vi "OAT Easy Continuous Resampling (Digital Tach).vi"(0 "scaled signal [EU]":waveform(dbl)={"t0"=timestamp(0 s since 1904-01-01), "dt"=0.0, "Y"=[]}, 1 "reset? (True)":bool=TRUE, 7 "digital tach info":T3={"tacho counts"=[], "counter timebase [Hz]"=20000000.0, "counter task type"=enum."event counting", "counter digit (32)"=32}, 9 "pulse/revolution (1)":i32=1, 11 "error in (no error)":errorcluster, 12 "max order (auto)":i32) -> (3 "speed profile":T1 {"speed [RPM]" format="%.2f"; "time [s]" format="%.2f"}, 4 "resampled signal":cluster{"r0":dbl, "dr":dbl, "Y":dbl[]} {"r0" format="%.2p"; "dr" format="%.2p"; "Y" format="%.2f"}, 6 "unit label":string, 10 "time instant":dbl[](array[numeric]) format="%.2f", 14 "channel info":T2={"sensor sensitivity [mV/EU]"=1000.0, "engineering units"=enum."V", "dB reference [EU]"=1.0, "custom label"="EU", "weighting filter"=enum."Linear", "pregain [dB]"=0.0} {"pregain [dB]" format="%.2f"; "dB reference [EU]" format="%.1e"; "sensor sensitivity [mV/EU]" format="%.2f"}, 15 "error out":errorcluster)   [LabVIEW 2017]
doc: "Resamples the even time-sampled <B>scaled signal [EU]</B> to an even angle-sampled signal. You can use this polymorphic VI to resample an analog tachometer signal or a digital tachometer signal. The data type you wire to the <B>analog tach signal</B> input determines the polymorphic instance to use."
uses:
  <vilib>/addons/Sound and Vibration/Order Analysis/Tach Process/SubVIs/digital tach info.ctl
  <vilib>/addons/Sound and Vibration/Order Analysis/Tach Process/SubVIs/speed profile.ctl
  <vilib>/addons/Sound and Vibration/Order Analysis/Backward Compatibility/OAT Resample Waveform (Single Channel).vi
  <vilib>/addons/Sound and Vibration/Order Analysis/Tach Process/SoundVib_TachProcess.lvlib
panel:
  # "OAT Easy Continuous Resampling (Digital Tach)"
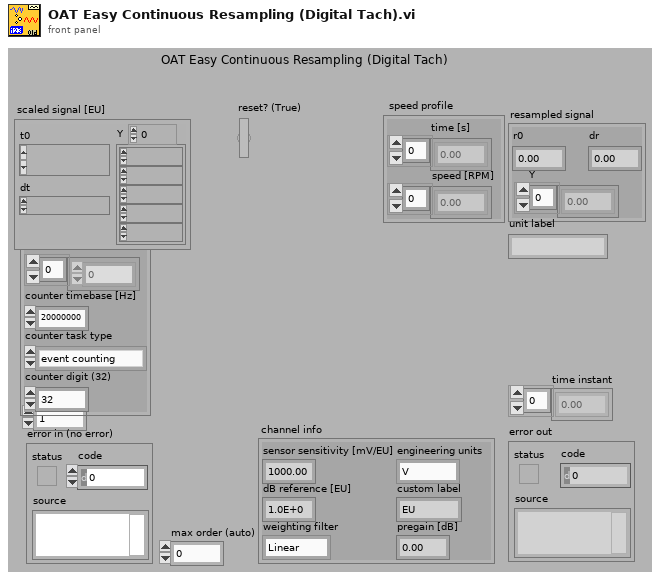
[diagram p1: front panel]
types:
  T1 = typedef "SoundVib_TachProcess.lvlib/speed profile.ctl" = cluster{"time [s]":dbl[], "speed [RPM]":dbl[]}
  T2 = cluster{"sensor sensitivity [mV/EU]":dbl, "engineering units":enum16{"custom...", "V", "Pa", "g", "m/s^2", "m/s", "m", "in/s^2", "in/s", "in"}, "dB reference [EU]":dbl, "custom label":string, "weighting filter":enum16{"Linear", "A-weighting", "B-weighting", "C-weighting"}, "pregain [dB]":dbl}
  T3 = typedef "SoundVib_TachProcess.lvlib/digital tach info.ctl" = cluster{"tacho counts":i64[], "counter timebase [Hz]":dbl, "counter task type":enum16{"period measurement", "event counting"}, "counter digit (32)":i32}
  T4 = typedef "svc_Channel Info.ctl" = cluster{"sensor sensitivity":dbl, "engineering units":T5, "dB reference":dbl, "custom label":string, "weighting filter":T6, "pregain":dbl}
  T5 = typedef "svc_Engineering Units Text Ring.ctl" = u16
  T6 = typedef "svc_Weighting Filter Text Ring.ctl" = u16
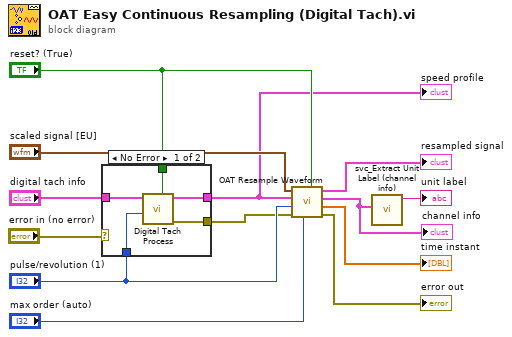
[diagram p0: block diagram]
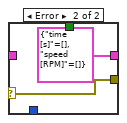
[diagram p2: hidden frame]
diagram:
  n1 = case shown="No Error" "error in (no error)" {
    selector: "error in (no error)" -> [_ w19]
    tunnel: "digital tach info" -> [w18 _]
    tunnel: "pulse/revolution (1)" -> [w17 _]
    tunnel: "reset? (True)" -> [w16 _]
    tunnel: [w15 T1 {"time [s]"=[], "speed [RPM]"=[]} ("speed profile")] -> w7
    tunnel: [w14 w19] -> w1
    frame No Error {
      n2 = call <vilib>:"Digital Tach Process.vi"("reset? (True)"=w16, "pulse/revolution (1)"=w17, "digital tach info"=w18) -> ("error out"=w14:errorcluster, "speed profile"=w15:T1)  [unwired: 6 in, 1 out]
    }
    frame Error {
    }
  }
  "speed profile" <- w7
  n3 = call-poly <vilib>:"OAT Resample Waveform.vi"("reset? (True)"="reset? (True)", "max order (auto)"="max order (auto)", "error in (no error)"=w1, "pulse/revolution (1)"="pulse/revolution (1)", "speed profile"=w7, "scaled signal [EU]"="scaled signal [EU]") -> ("error out"=→"error out":errorcluster, "interpolated pulse positions"=→"time instant":dbl[], "channel info"=w6:T4, "resampled signal"=→"resampled signal":cluster{"r0":dbl, "dr":dbl, "Y":dbl[]})  [unwired: 2 in]
  "channel info" <- w6
  n4 = call <vilib>:"svc_Extract Unit Label (channel info).vi"("channel info"=w6) -> ("unit label"=→"unit label":string)  [unwired: 8 in, 2 out]
